vi "close.vi"(8 "error in (no error)":errorcluster, 11 "NEXUS in":refnum<class "NEXUS.lvclass">) -> (0 "error out":errorcluster, 3 "NEXUS out":refnum<class "NEXUS.lvclass">)   [LabVIEW 2019, in "NEXUS.lvclass"]
uses:
  NEXUS.lvclass
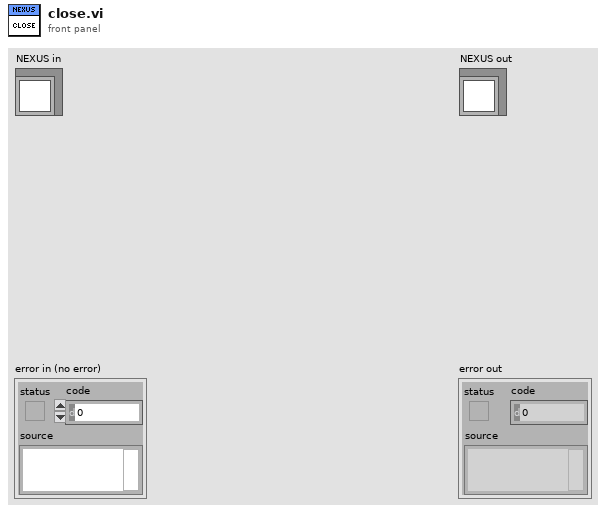
[diagram p1: front panel]
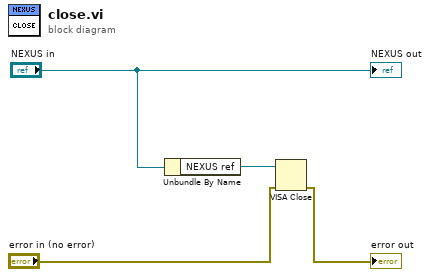
[diagram p0: block diagram]
diagram:
  n1 = Unbundle By Name("NEXUS in") -> ("NEXUS ref"=w4:refnum<visa-resource-name>)
  n2 = VISA Close(VISA resource name=w4, error in (no error)="error in (no error)") -> (error out=→"error out":errorcluster)
  "NEXUS out" <- "NEXUS in"
